vi "test event queue.vi"() -> ()   [LabVIEW 2013, in "tag bus tests.lvlib"]
uses:
  tag bus tests.lvlib
  events/event.ctl
  events/data bus events.lvlib
panel:
  out "overflow OK 2":bool
  out "not overflow OK 2":bool
  out "not overflow OK":bool
  out "overflow OK":bool
  out "load ok":bool
  out "init ok":bool
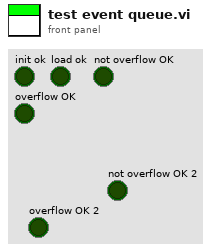
[diagram p1: front panel]
types:
  T1 = typedef "data bus events.lvlib/event queue.ctl" = cluster{"queues":T2[]}
  T2 = typedef "data bus events.lvlib/event queue element.ctl" = cluster{"head":i32, "count":i32, "event array":T3[]}
  T3 = typedef "data bus events.lvlib/event.ctl" = cluster{"event group":i64, "event ID":i64, "int value":i64, "double value":dbl, "event time":timestamp}
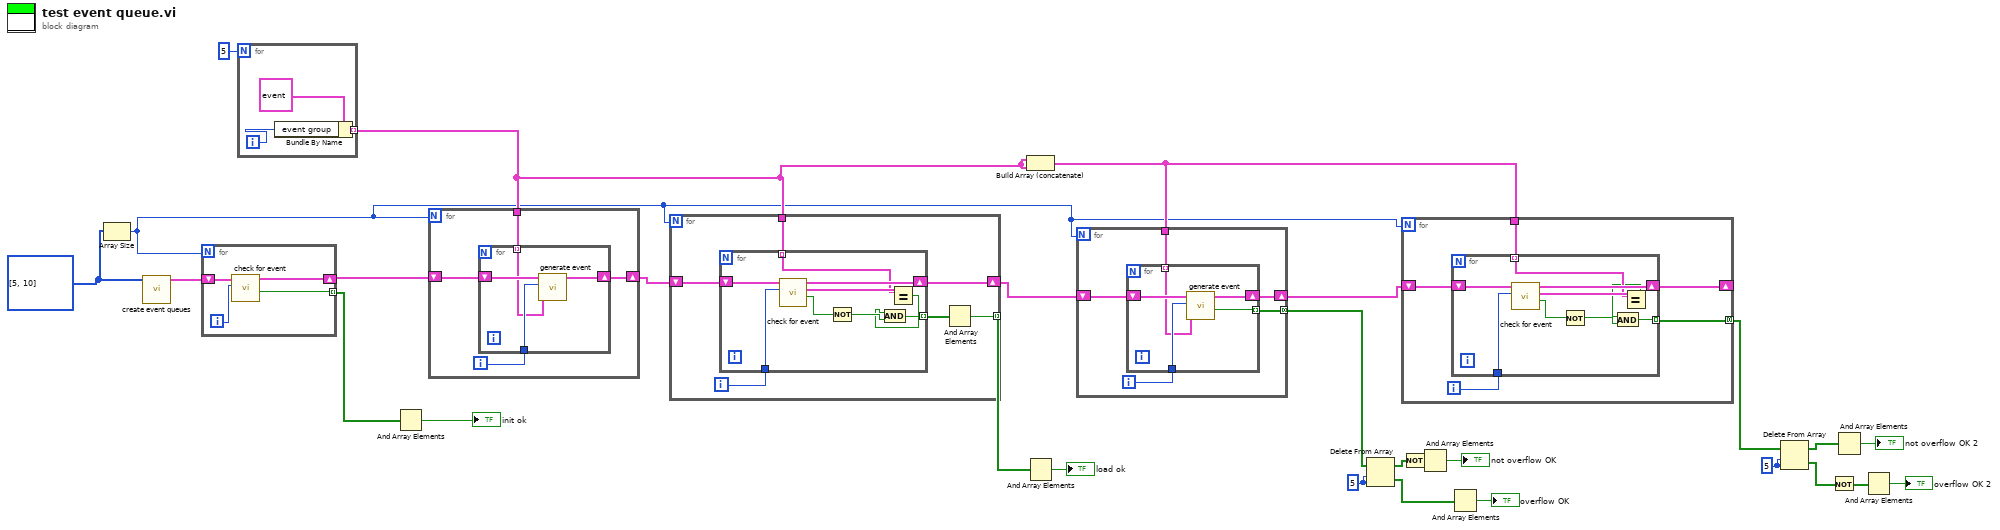
[diagram p0: block diagram]
diagram:
  w5 = 5 ("index")
  w16 = 5 ("index")
  w28 = i32[] [5, 10] ("sizes")
  n1 = Array Size(array=w28) -> (size(s)=w3:i32)
  n2 = call "create event queues.vi"("sizes"=w28) -> ("event queue"=w27:T1)  [unwired: 10 in]
  n3 = for {
    N: w3 -> [_]
    shift-right: [w30] -> w24
    shift-left: w27 -> [w31]
    tunnel: [w29] -> w26 mode=indexing
    i -> [w32]
    n4 = call "check for event.vi"("queue index"=w32, "event queue in"=w31) -> ("empty?"=w29:bool, "event queue out"=w30:T1)  [unwired: 7 in, 1 out]
  }
  n5 = for {
    N: 5 -> [_]
    tunnel: [w33] -> w19 mode=indexing
    i -> [w34]
    n6 = Bundle By Name(cluster=T3 {"event group"=0, "event ID"=0, "int value"=0, "double value"=0.0, "event time"=timestamp(0 s since 1904-01-01)} ("event"), "event group"=w34) -> (w33:T3)
  }
  n7 = And Array Elements(Boolean array=w26) -> (logical AND=→"init ok":bool)
  n8 = for {
    N: w3 -> [_]
    shift-right: [w37] -> w22
    shift-left: w24 -> [w38]
    tunnel: w19 -> [w36]
    i -> [w39]
    n9 = for {
      tunnel: w39 -> [w42]
      shift-right: [w41] -> w37
      shift-left: w38 -> [w43]
      tunnel: w36 -> [w40] mode=indexing
      n10 = call "generate event.vi"("event"=w40, "queue index"=w42, "event queue in"=w43) -> ("event queue out"=w41:T1)  [unwired: 7 in, 1 out]
    }
  }
  n11 = for {
    N: w3 -> [_]
    shift-right: [w47] -> w18
    shift-left: w22 -> [w48]
    tunnel: w19 -> [w46]
    tunnel: [w44] -> w21 mode=indexing
    i -> [w49]
    n12 = for {
      tunnel: w49 -> [w57]
      shift-right: [w56] -> w47
      shift-left: w48 -> [w58]
      tunnel: w46 -> [w54] mode=indexing
      tunnel: [w50] -> w45 mode=indexing
      n13 = call "check for event.vi"("queue index"=w57, "event queue in"=w58) -> ("empty?"=w53:bool, "event"=w55:T3, "event queue out"=w56:T1)  [unwired: 7 in]
      n14 = Not(x=w53) -> (.not. x?=w52:bool)
      n15 = Equal?(x=w54, y=w55) -> (x = y?=w51:bool)
      n16 = And(x=w51, y=w52) -> (x .and. y?=w50:bool)
    }
    n17 = And Array Elements(Boolean array=w45) -> (logical AND=w44:bool)
  }
  n18 = Build Array (concatenate)(w19, w19) -> (w9:T3[])
  n19 = And Array Elements(Boolean array=w21) -> (logical AND=→"load ok":bool)
  n20 = for {
    N: w3 -> [_]
    shift-right: [w61] -> w10
    shift-left: w18 -> [w62]
    tunnel: w9 -> [w60]
    tunnel: [w59] -> w17 mode=concatenating
    i -> [w63]
    n21 = for {
      tunnel: w63 -> [w67]
      shift-right: [w66] -> w61
      shift-left: w62 -> [w68]
      tunnel: w60 -> [w65] mode=indexing
      tunnel: [w64] -> w59 mode=indexing
      n22 = call "generate event.vi"("event"=w65, "queue index"=w67, "event queue in"=w68) -> ("failed?"=w64:bool, "event queue out"=w66:T1)  [unwired: 7 in]
    }
  }
  n23 = Delete From Array(array=w17, length=w16, index=w16) -> (deleted portion=w11:bool[], array with subset deleted=w15:bool[])
  n24 = Not(x=w15) -> (.not. x?=w12:bool[])
  n25 = for {
    N: w3 -> [_]
    shift-right: [w71] -> _
    shift-left: w10 -> [w72]
    tunnel: w9 -> [w70]
    tunnel: [w69] -> w4 mode=concatenating
    i -> [w73]
    n26 = for {
      tunnel: w73 -> [w81]
      shift-right: [w80] -> w71
      shift-left: w72 -> [w82]
      tunnel: w70 -> [w78] mode=indexing
      tunnel: [w74] -> w69 mode=indexing
      n27 = call "check for event.vi"("queue index"=w81, "event queue in"=w82) -> ("empty?"=w77:bool, "event"=w79:T3, "event queue out"=w80:T1)  [unwired: 7 in]
      n28 = Not(x=w77) -> (.not. x?=w76:bool)
      n29 = Equal?(x=w78, y=w79) -> (x = y?=w75:bool)
      n30 = And(x=w75, y=w76) -> (x .and. y?=w74:bool)
    }
  }
  n31 = And Array Elements(Boolean array=w12) -> (logical AND=→"not overflow OK":bool)
  n32 = And Array Elements(Boolean array=w11) -> (logical AND=→"overflow OK":bool)
  n33 = Delete From Array(array=w4, length=w5, index=w5) -> (deleted portion=w8:bool[], array with subset deleted=w2:bool[])
  n34 = Not(x=w8) -> (.not. x?=w1:bool[])
  n35 = And Array Elements(Boolean array=w2) -> (logical AND=→"not overflow OK 2":bool)
  n36 = And Array Elements(Boolean array=w1) -> (logical AND=→"overflow OK 2":bool)
